vi "Main.vi"() -> ()   [LabVIEW 2021]
uses:
  System.Windows.Forms
  tdefs/td.Message.ctl
  tdefs/td.SensorCheck.ctl
panel:
  in  "Event Structure":bool
  in  "btn.Stop":bool
  in  "Max Level 2":dbl(slide) scale=0.0..10.0
  in  "Max Level 1":dbl(slide) scale=0.0..10.0
  in  "Emergency 2":dbl(slide) scale=0.0..10.0
  in  "Emergency 1":dbl(slide) scale=0.0..10.0
  out "Time Stamp 2":timestamp
  out "Time Stamp":timestamp
  in  "DateTimePicker 2":refnum<k24>(container)
  in  "DateTimePicker":refnum<k24>(container)
  out "Command":string
  out "Log":string
  out "Time":string
  # "can be headless so all callbacks"
  # "Alerts"
  # "Example .net"
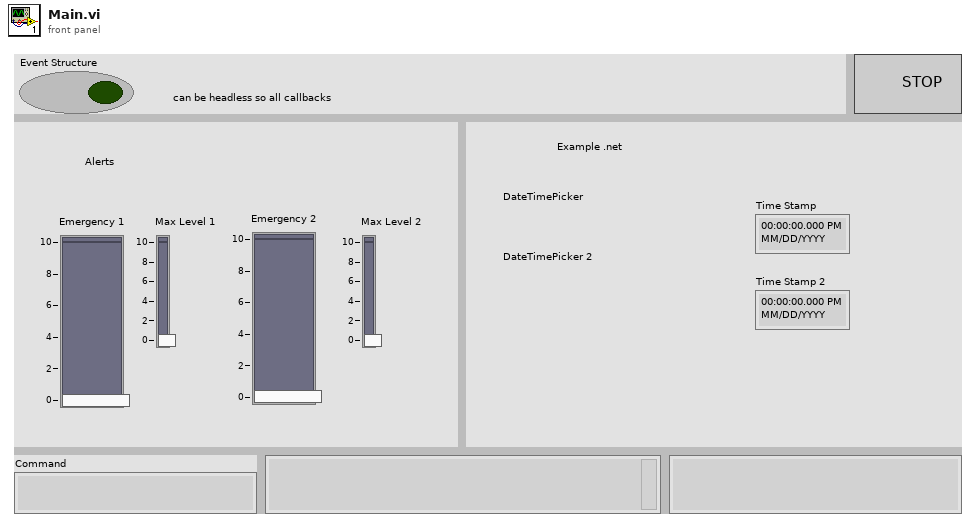
[diagram p1: front panel]
types:
  T1 = typedef "td.SensorCheck.ctl" = cluster{"Max Lim":refnum<vi>, "queue Ref":refnum<queue>}
  T2 = typedef "td.Message.ctl" = cluster{"Command":string, "Data":variant}
  T3 = cluster{"Stop":refnum<user-event>, "Time":refnum<user-event>, "Time2":refnum<user-event>}
  T4 = cluster{"Time":refnum<user-event>, "queue out":refnum<queue>}
  T5 = cluster{"Time2":refnum<user-event>, "queue out":refnum<queue>}
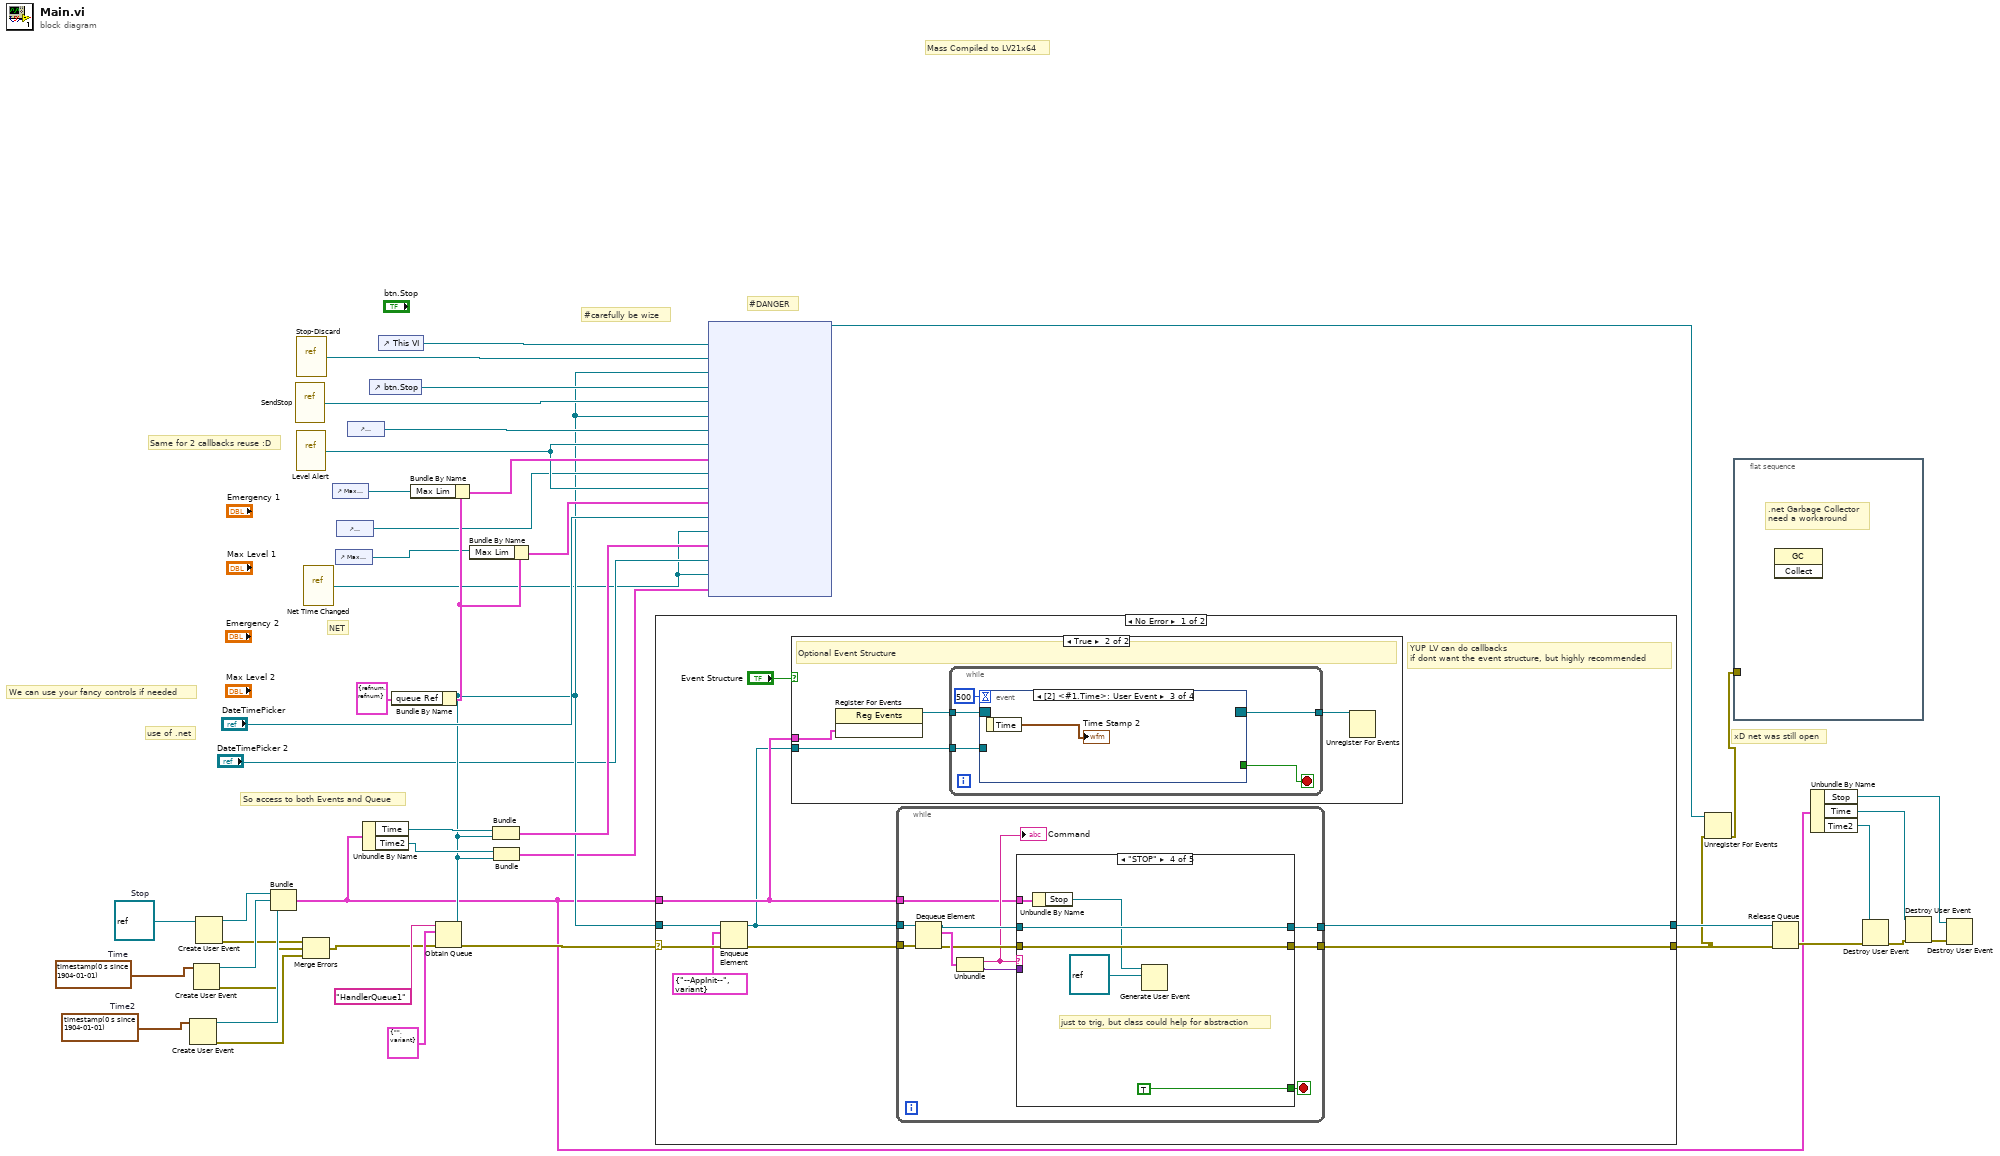
[diagram p0: block diagram]
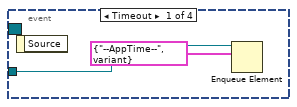
[diagram p3: hidden frame]
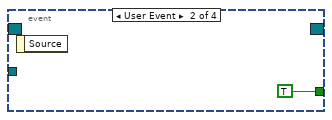
[diagram p4: hidden frame]
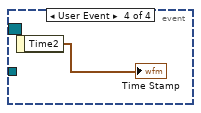
[diagram p5: hidden frame]
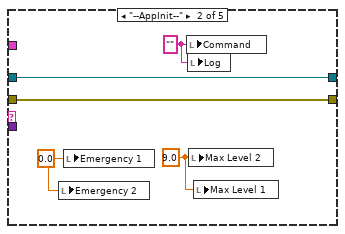
[diagram p7: hidden frame]
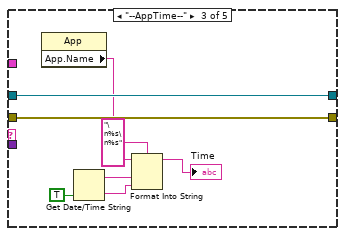
[diagram p8: hidden frame]
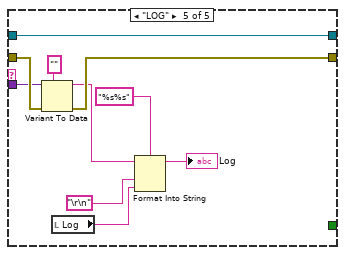
[diagram p9: hidden frame]
diagram:
  w25 = timestamp(0 s since 1904-01-01)  # Time2
  w26 = timestamp(0 s since 1904-01-01)  # Time
  w27 = refnum<class> refnum  # Stop
  # "Mass Compiled to LV21x64"
  # "xD net was still open"
  # "NET"
  # "#DANGER"
  # "We can use your fancy controls if needed"
  # "use of .net"
  # "So access to both Events and Queue"
  # "Same for 2 callbacks reuse :D"
  # "#carefully be wize"
  n1 = Create User Event(user event datatype=w25) -> (user event=w22:refnum<user-event>, error out=w19:errorcluster)  [unwired: 1 in]
  n2 = Create User Event(user event datatype=w26) -> (user event=w23:refnum<user-event>, error out=w20:errorcluster)  [unwired: 1 in]
  n3 = Create User Event(user event datatype=w27) -> (user event=w24:refnum<user-event>, error out=w21:errorcluster)  [unwired: 1 in]
  n4 = Bundle("Stop"=w24, "Time"=w23, "Time2"=w22) -> (w7:T3)  [unwired: 1 in]
  n5 = vi-ref "SendStop.vi"() -> ("vi reference"=w38:refnum<vi>)
  n6 = vi-ref "Level Alert.vi"() -> ("vi reference"=w30:refnum<vi>)
  n7 = vi-ref "Stop-Discard.vi"() -> ("vi reference"=w40:refnum<vi>)
  n8 = Merge Errors(w21, w20, w19) -> (w18:errorcluster)
  n9 = vi-ref "Net Time Changed.vi"() -> ("vi reference"=w11:refnum<vi>)
  n10 = control-ref of="Max Level 1"() -> (w35:refnum<vi>)
  n11 = control-ref of="Max Level 2"() -> (w34:refnum<vi>)
  n12 = control-ref of="Emergency 2"() -> (w29:refnum<vi>)
  n13 = control-ref of="Emergency 1"() -> (w33:refnum<vi>)
  n14 = Unbundle By Name(w7) -> ("Time"=w16:refnum<user-event>, "Time2"=w15:refnum<user-event>)
  n15 = control-ref of="btn.Stop"() -> (w39:refnum<vi>)
  n16 = control-ref of="This VI"() -> (w41:refnum<vi>)
  n17 = Obtain Queue(name (unnamed)="HandlerQueue1", element data type=T2 {"Command"="", "Data"=variant} ("Message"), error in (no error)=w18) -> (queue out=w14:refnum<queue>, error out=w43:errorcluster)  [unwired: 2 in, 1 out]
  n18 = Bundle By Name(cluster=T1 {"Max Lim"=refnum, "queue Ref"=refnum} ("SensorCheck"), "queue Ref"=w14) -> (w36:T1)
  n19 = Bundle By Name(cluster=w36, "Max Lim"=w35) -> (w32:T1)
  n20 = Bundle By Name(cluster=w36, "Max Lim"=w34) -> (w31:T1)
  n21 = Bundle("Time"=w16, "queue out"=w14) -> (w17:T4)  [unwired: 1 in]
  n22 = Bundle("Time2"=w15, "queue out"=w14) -> (w12:T5)  [unwired: 1 in]
  n23 = case shown="No Error" w43 {
    selector: w43 -> [w51 w111]
    tunnel: w14 -> [w54 w112]
    tunnel: [w53 w112] -> w42
    tunnel: [w52 w111] -> w3
    tunnel: w7 -> [w47 _]
    frame No Error {
      # "YUP LV can do callbacks\nif dont want the event structure, but highly recommended"
      n24 = Enqueue Element(queue=w54, element=T2 {"Command"="--AppInit--", "Data"=variant}, error in (no error)=w51) -> (queue out=w46:refnum<queue>, error out=w50:errorcluster)  [unwired: 1 in, 1 out]
      n25 = case shown="True" "Event Structure" {
        tunnel: w47 -> [_ w56]
        tunnel: w46 -> [_ w55]
        frame False {
        }
        frame True {
          # "Optional Event Structure"
          n26 = register-events(w56) -> (reference out=w58:refnum<event-registration>)  [unwired: 2 in, 1 out]
          n27 = while {
            tunnel: w58 -> [w63]
            tunnel: [w62] -> w57
            tunnel: w55 -> [w61]
            stop <- w59 stop-if-true
            n28 = event shown="[2] <#1.Time>: User Event" {
              selector: w63 -> [_ _ _ _]
              dyn-events: [_ _ _ _] -> w62
              timeout: 500 -> [_ _ _ _]
              tunnel: w61 -> [w65 _ _ _]
              tunnel: [_ TRUE _ _] -> w59
              event Timeout {
                n29 = event-data() -> ()  [unwired: 1 in, 1 out]
                n30 = Enqueue Element(queue=w65, element=T2 {"Command"="--AppTime--", "Data"=variant}) -> ()  [unwired: 2 in, 3 out]
              }
              event User Event {
                n31 = event-data() -> ()  [unwired: 1 in, 1 out]
              }
              event User Event {
                n32 = event-data() -> ("Time"=→"Time Stamp 2":timestamp)  [unwired: 1 in]
              }
              event User Event {
                n33 = event-data() -> ("Time2"=→"Time Stamp":timestamp)  [unwired: 1 in]
              }
            }
          }
          n34 = Unregister For Events(event registration refnum=w57) -> ()  [unwired: 1 in, 1 out]
        }
      }
      n35 = while {
        tunnel: w46 -> [w79]
        tunnel: w50 -> [w76]
        tunnel: [w74] -> w53
        tunnel: [w72] -> w52
        tunnel: w47 -> [w69]
        stop <- w71 stop-if-true
        n36 = Dequeue Element(queue=w79, error in (no error)=w76) -> (queue out=w73:refnum<queue>, element=w78:T2, error out=w75:errorcluster)  [unwired: 1 in, 1 out]
        n37 = Unbundle(w78) -> ("Command"=w70:string, "Data"=w77:variant)
        "Command" <- w70
        n38 = case shown="\"STOP\"" w70 {
          tunnel: w77 -> [_ _ _ _ w107]
          tunnel: w75 -> [w80 w85 w93 w99 w109]
          tunnel: [w81 w86 w94 w100 w110] -> w74
          tunnel: w73 -> [w81 w86 w94 w100 w110]
          tunnel: [w80 w85 w93 w99 w108] -> w72
          tunnel: [_ _ _ TRUE _] -> w71
          tunnel: w69 -> [_ _ _ w97 _]
          frame Default {
          }
          frame "--AppInit--" {
            w82 = 0.0 ("Emergency 1")
            w83 = 9.0 ("Max Level 2")
            w84 = "" ("Command")
            n39 = local write "Emergency 2"(w82) -> ()
            n40 = local write "Emergency 1"(w82) -> ()
            n41 = local write "Command"(w84) -> ()
            n42 = local write "Log"(w84) -> ()
            n43 = local write "Max Level 2"(w83) -> ()
            n44 = local write "Max Level 1"(w83) -> ()
          }
          frame "--AppTime--" {
            n45 = property class="App"() -> ("App.Name"=w88:string)  [unwired: 2 in, 2 out]
            n46 = Get Date/Time String(want seconds? (F)=TRUE) -> (date string=w90:string, time string=w89:string)  [unwired: 2 in]
            n47 = Format Into String(format string="\n%s\n%s", initial string=w88, w90, w89) -> (resulting string=→"Time":string)  [unwired: 1 in, 1 out]
          }
          frame "STOP" {
            # "just to trig, but class could help for abstraction"
            n48 = Unbundle By Name(w97) -> ("Stop"=w96:refnum<user-event>)
            n49 = Generate User Event(user event=w96, event data cluster=refnum<class> refnum ("event data")) -> ()  [unwired: 2 in, 2 out]
          }
          frame "LOG" {
            n50 = Variant To Data(error in=w109, type="" ("format string"), Variant=w107) -> (data=w104:string, error out=w108:errorcluster)
            n51 = local read "Log"() -> (w101:string)
            n52 = Format Into String(format string="%s%s", initial string=w104, "\r\n", w101) -> (resulting string=→"Log":string)  [unwired: 1 in, 1 out]
          }
        }
      }
    }
    frame Error {
    }
  }
  n53 = node(w41, w40, w14, w39, w38, w14, w33, w30, w32, w29, w30, w31, "DateTimePicker", w11, w17, "DateTimePicker 2", w11, w12) -> (w1:refnum<k27>)  [unwired: 2 in, 1 out]
  n54 = Unregister For Events(event registration refnum=w1, error in=w3) -> (error out=w2:errorcluster)
  n55 = flat-sequence {
    tunnel: w2 -> [_]
    frame #0 {
      # ".net Garbage Collector\nneed a workaround"
      n56 = invoke class="GC" method="Collect"() -> ()  [unwired: 3 in, 3 out]
    }
  }
  n57 = Release Queue(queue=w42, error in (no error)=w3) -> (error out=w10:errorcluster)  [unwired: 1 in, 2 out]
  n58 = Unbundle By Name(w7) -> ("Stop"=w4:refnum<user-event>, "Time"=w5:refnum<user-event>, "Time2"=w6:refnum<user-event>)
  n59 = Destroy User Event(user event=w6, error in=w10) -> (error out=w8:errorcluster)
  n60 = Destroy User Event(user event=w5, error in=w8) -> (error out=w9:errorcluster)
  n61 = Destroy User Event(user event=w4, error in=w9) -> ()  [unwired: 1 out]
